vi "stepper.vi"() -> ()   [LabVIEW 2015]
doc: "This example shows a single axis straight line move using an ISM or SMD Ethernet drive. \n\nNote: You must have the LabVIEW NI SoftMotion Module installed to run this example."
uses:
  <vilib>/Motion/PropertyNodes/nimc.createStraightLineMoveInstance.axis.vi
  <vilib>/Motion/PropertyNodes/nimc.destroyInterfaceInstance.vi
  <resource>/objmgr/nimotion.rc
  <resource>/objmgr/nimcca.rc
panel:
  in  "Smoothing":dbl
  in  "Deccel Jerk":dbl
  in  "Acceleration Jerk":dbl
  out "Speed":dbl(knob) scale=0.0..5000.0
  out "Waveform Chart":dbl(graph)
  in  "Enable":bool
  in  "Axis":refnum<k21>="niss://192.168.1.10"
  in  "Deceleration":dbl
  out "error out":errorcluster
  in  "Move Mode":i32(ring)=10551344 items=["Absolute"=10551337, "Relative"=10551344, "Relative To Capture"=10551345, "Velocity"=10551346]
  out "?":dbl(graph)
  in  "Acceleration":dbl=7200.0
  in  "Velocity":dbl=60.0
  in  "Position":dbl=6000.0
  in  "Stop Move":bool
  in  "Start Move":bool
  in  "stop":bool
  # "Move Constraints"
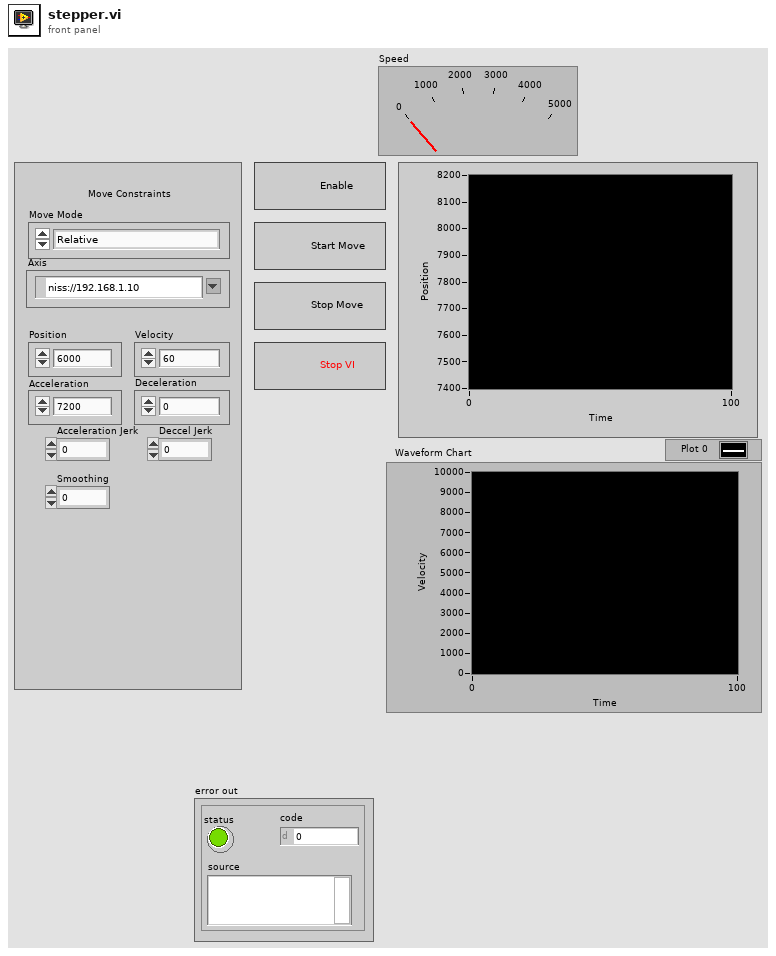
[diagram p1: front panel]
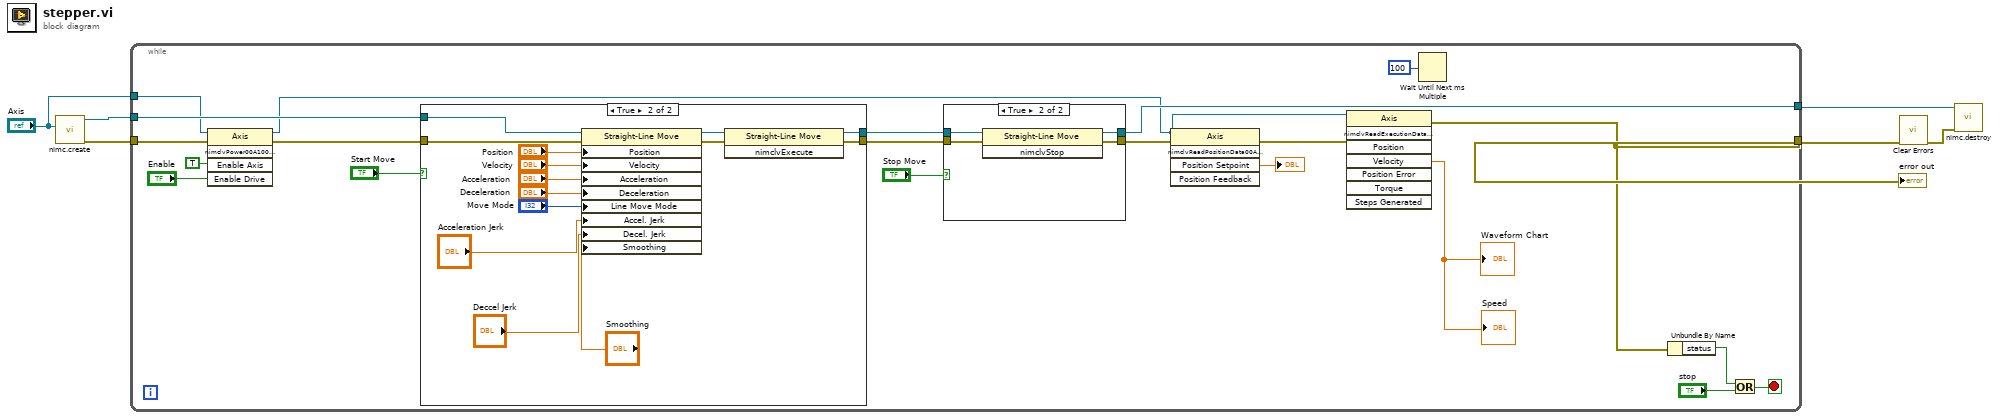
[diagram p0: block diagram]
diagram:
  n1 = call-poly <vilib>:"nimc.create.vi"("axis"="Axis") -> ("error out"=w5:errorcluster, "line"=w6:refnum<k20>)  [unwired: 8 in, 1 out]
  n2 = while {
    tunnel: w6 -> [w27]
    tunnel: w5 -> [w15]
    tunnel: "Axis" -> [w13]
    tunnel: [w9] -> w2
    tunnel: [w17] -> w4
    stop <- w19 stop-if-true
    n3 = invoke class="Axis" method="nimclvPower00A10001"(reference=w13, error in=w15, "Enable Axis"=TRUE, "Enable Drive"="Enable") -> (reference out=w10:refnum<k21>, error out=w14:errorcluster)  [unwired: 1 in, 3 out]
    n4 = case shown="True" "Start Move" {
      tunnel: w27 -> [w35 w49]
      tunnel: w14 -> [w34 w46]
      tunnel: [w34 w45] -> w22
      tunnel: [w35 w44] -> w21
      frame False {
      }
      frame True {
        n5 = property class="Straight-Line Move"(reference=w49, error in=w46, "Position"="Position", "Velocity"="Velocity", "Acceleration"="Acceleration", "Deceleration"="Deceleration", "Line Move Mode"="Move Mode", "Accel. Jerk"="Acceleration Jerk", "Decel. Jerk"="Deccel Jerk", "Smoothing"="Smoothing") -> (reference out=w48:refnum<k20>, error out=w47:errorcluster)
        n6 = invoke class="Straight-Line Move" method="nimclvExecute"(reference=w48, error in=w47) -> (reference out=w44:refnum<k20>, error out=w45:errorcluster)  [unwired: 1 in, 1 out]
      }
    }
    n7 = case shown="True" "Stop Move" {
      tunnel: w22 -> [w29 w32]
      tunnel: w21 -> [w28 w33]
      tunnel: [w29 w31] -> w20
      tunnel: [w28 w30] -> w17
      frame False {
      }
      frame True {
        n8 = invoke class="Straight-Line Move" method="nimclvStop"(reference=w33, error in=w32) -> (reference out=w30:refnum<k20>, error out=w31:errorcluster)  [unwired: 1 in, 1 out]
      }
    }
    n9 = invoke class="Axis" method="nimclvReadPositionData00A10001"(reference=w10, error in=w20) -> (error out=w8:errorcluster, "Position Setpoint"=→"?":dbl)  [unwired: 3 in, 3 out]
    n10 = invoke on="Invoke Node" class="Axis" method="nimclvReadExecutionData00A10001"(reference=w10, error in=w8) -> (error out=w9:errorcluster, "Velocity"=→"Waveform Chart" →"Speed":dbl)  [unwired: 6 in, 6 out]
    n11 = Wait Until Next ms Multiple(millisecond multiple=u32 100 ("milliseconds to wait")) -> ()  [unwired: 1 out]
    n12 = Unbundle By Name(w9) -> ("status"=w18:bool)
    n13 = Or(x=w18, y="stop") -> (x .or. y?=w19:bool)
  }
  "error out" <- w2
  n14 = call <vilib>:"Clear Errors.vi"("error in (no error)"=w2) -> ("error out"=w3:errorcluster)  [unwired: 5 in, 1 out]
  n15 = call-poly <vilib>:"nimc.destroy.vi"("error in"=w3, "motion handle"=w4) -> ()  [unwired: 9 in, 1 out]
